vi "ReCalcAnimator.vi"(0 "Image Array":T1[](array[typedef]), 7 "Pict Refnum":refnum<vi>, 11 "error in (no error)":errorcluster) -> (4 "Pic Array":picture[](array[picture]), 15 "error out":errorcluster)   [LabVIEW 2019, in "AnimatorXControl.xctl"]
uses:
  AnimatorXControl.xctl
  <vilib>/picture/picture.llb/imagedata.ctl
  DefaultImageData.vi
panel:
  out "Picture":picture
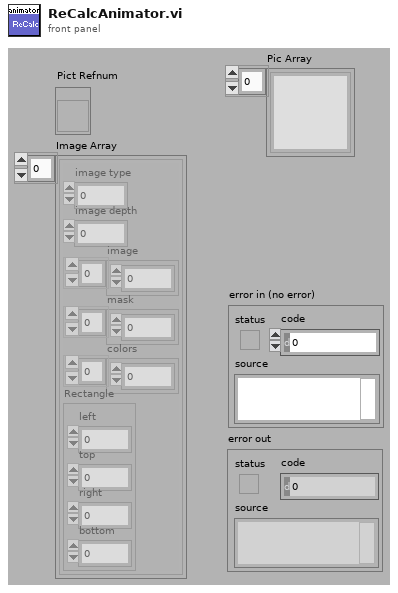
[diagram p1: front panel]
types:
  T1 = typedef "imagedata.ctl" = cluster{"image type":i32, "image depth":i32, "image":u8[], "mask":u8[], "colors":u32[], "Rectangle":cluster{"left":i16, "top":i16, "right":i16, "bottom":i16}}
  T2 = typedef "LVPointTypeDef.ctl" = cluster{"Horizontal":i16, "Vertical":i16}
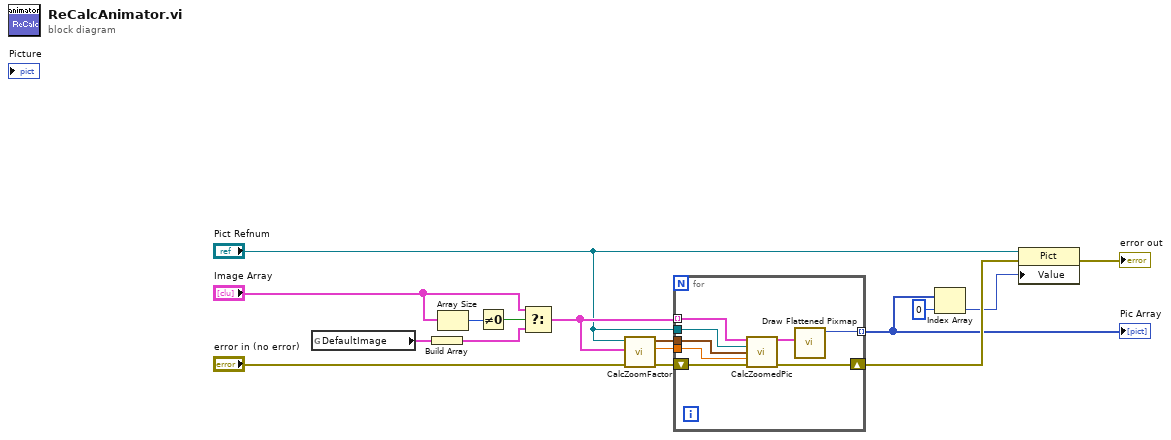
[diagram p0: block diagram]
diagram:
  n1 = global read "DefaultImageData.vi" "DefaultImage"() -> (w15:T1)
  n2 = Build Array(w15) -> (w14:T1[])
  n3 = Array Size(array="Image Array") -> (size(s)=w16:i32)
  n4 = Not Equal To 0?(x=w16) -> (x != 0?=w13:bool)
  n5 = Select(t="Image Array", s=w13, f=w14) -> (s? t:f=w5:T1[])
  n6 = call "CalcZoomFactor.vi"("error in (no error)"="error in (no error)", "Image Array"=w5, "Pict Refnum"="Pict Refnum") -> ("error out"=w10:errorcluster, "ZoomFactor"=w7:dbl, "OriginPoint"=w6:T2)  [unwired: 6 in]
  n7 = for {
    tunnel: w7 -> [w22]
    tunnel: w6 -> [w21]
    tunnel: w5 -> [w20] mode=indexing
    tunnel: [w18] -> w3 mode=indexing
    shift-right: [w23] -> w9
    shift-left: w10 -> [w24]
    tunnel: "Pict Refnum" -> [w17]
    n8 = call "CalcZoomedPic.vi"("Image Data In"=w20, "Pict Refnum"=w17, "OriginPoint"=w21, "ZoomFactor"=w22, "error in (no error)"=w24) -> ("Image Data Out"=w19:T1, "error out"=w23:errorcluster)  [unwired: 9 in]
    n9 = call <vilib>:"Draw Flattened Pixmap.vi"("image data"=w19) -> ("new picture"=w18:picture)  [unwired: 8 in]
  }
  "Pic Array" <- w3
  n10 = Index Array(array=w3, index=0) -> (element=w1:picture)
  n11 = property class="Pict"(reference="Pict Refnum", error in=w9, "Value"=w1) -> (error out=→"error out":errorcluster)  [unwired: 1 out]
